vi "stopVideo.vi"(8 "error in (no error)":errorcluster, 11 "AtomChipHWC in":refnum<class "AtomChipHWC.lvclass">) -> (0 "error out":errorcluster, 3 "AtomChipHWC out":refnum<class "AtomChipHWC.lvclass">)   [LabVIEW 2009, in "Hardware.lvlib" / "HWControllers.lvlib" / "AtomChipHWC.lvclass"]
uses:
  AtomChipHWC.lvclass
  HardwareConfiguration/HWConfiguration.lvclass
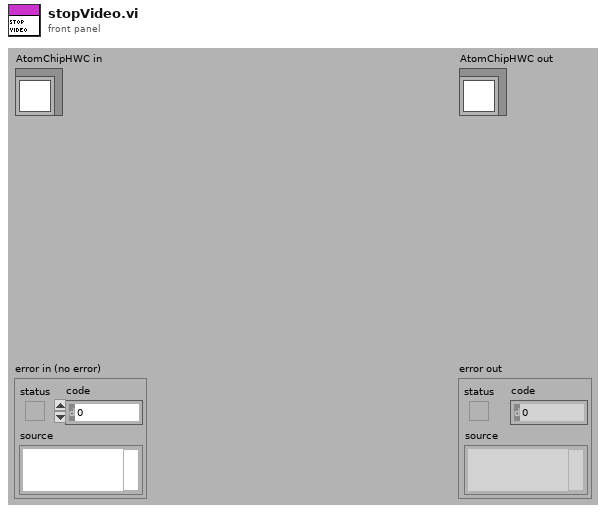
[diagram p1: front panel]
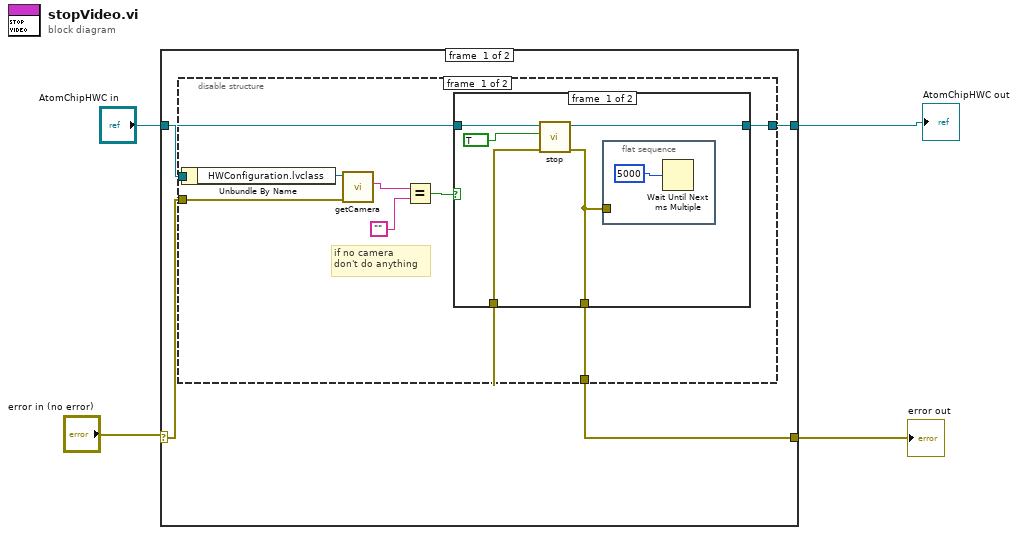
[diagram p0: block diagram]
diagram:
  n1 = case shown="No Error" "error in (no error)" {
    selector: "error in (no error)" -> [w5 w27]
    tunnel: [w8 w28] -> w3
    tunnel: "AtomChipHWC in" -> [w6 w28]
    tunnel: [w7 w27] -> w1
    frame #0 {
      n2 = disable-structure shown="Enabled" {
        disable-tunnel: [w16 w26] -> w8
        disable-tunnel: [w15 w25] -> w7
        disable-tunnel: w6 -> [w13 w26]
        disable-tunnel: w5 -> [w12 w25]
        frame #0 {
          # "if no camera\ndon't do anything"
          n3 = Unbundle By Name(w13) -> ("HWConfiguration.lvclass"=w14:refnum<class "HWConfiguration.lvclass">)
          n4 = call-dynamic "getCamera.vi"("error in (no error)"=w12, "HWConfiguration.lvclass in"=w14) -> ("camera"=w11:string)  [unwired: 7 in, 2 out]
          n5 = Equal?(x=w11, y="") -> (x = y?=w9:bool)
          n6 = case shown="True" w9 {
            tunnel: [w21 w24] -> w16
            tunnel: [w20 w23] -> w15
            tunnel: w13 -> [w19 w24]
            tunnel: w12 -> [w18 w23]
            frame #0 {
              n7 = call-dynamic "stop.vi"("error in (no error)"=w18, "stop?"=TRUE, "AtomChipHWC in"=w19) -> ("error out"=w20:errorcluster, "AtomChipHWC out"=w21:refnum<class "AtomChipHWC.lvclass">)  [unwired: 6 in, 1 out]
              n8 = flat-sequence {
                tunnel: w20 -> [_]
                frame #0 {
                  n9 = Wait Until Next ms Multiple(millisecond multiple=5000) -> ()  [unwired: 1 out]
                }
              }
            }
            frame #1 {
            }
          }
        }
        frame #1 {
        }
      }
    }
    frame #1 {
    }
  }
  "error out" <- w1
  "AtomChipHWC out" <- w3
